vi "AutomaticCalibration.vi"(8 "error in (no error)":errorcluster, 11 "Path":path) -> (0 "error out":errorcluster, 3 "Path Out":path)   [LabVIEW 2013, in "main.lvlib"]
uses:
  main.lvlib
  <vilib>/Analysis/6fits.llb/Curve Fitting Criteria.ctl
  Controls/Enum Save Action Events.ctl
  <vilib>/Analysis/1siggen.llb/Ramp Pattern by Samples.vi
  <userlib>/_OpenG.lib/file/file.llb/File Exists - Scalar__ogtk.vi
  Globals/DataAcqRecordPathGlobal.vi
  <vilib>/Analysis/NI_AAL_SigProc.lvlib
  <vilib>/Analysis/NI_AALBase.lvlib
  <vilib>/Analysis/NI_AALPro.lvlib
panel:
  out "Linear Fit":cluster{dbl[], "Best Linear Fit":dbl[]}[](graph)
  in  "CalibrationCancelBtn":bool
  in  "CalibrationStopBtn":bool
  in  "Slide":dbl(slide) scale=-0.6587369139847334..-0.5375357904577545 scale format="%#_2g"
  out "System XY Graph":cluster{"Ramp Pattern":dbl[], dbl[]}[](graph)
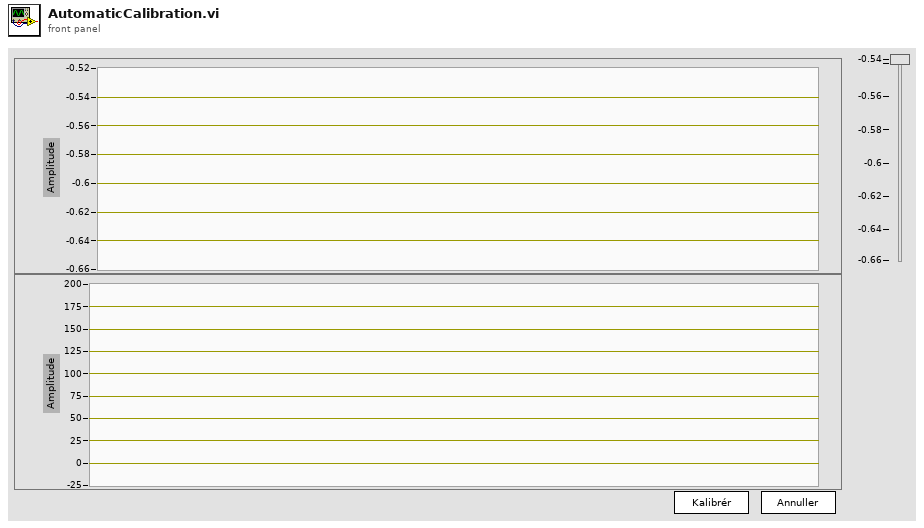
[diagram p1: front panel]
types:
  T1 = typedef "main.lvlib/Enum Save Action Events.ctl" = enum16{"LoadReportPath", "SaveReportPath", "Load Graph Path", "Save Graph Path", "LoadDataPath", "SaveDataPath", "Load Template Path", "Save Template Path", "Load PressureFactor", "Save PressureFactor", "Init", "Load Listbox", "Save Listbox", "LoadHospInfo", "SaveHospInfo", "Load DICOM Activation", "Save DICOM Activation", "LoadDICOMInfoWL", "SaveDICOMInfoWL", "LoadDICOMInfoPACS", "SaveDICOMInfoPACS", "Load ArmCalcMethod", "Save ArmCalcMethod", "LoadItemTags", "SaveItemTags", "LoadDICOMEncoding", "SaveDICOMEncoding", "LoadJournalType", "SaveJournalType", "LoadAcqFilterType", "SaveAcqFilterType", "Load Sequence", "Save Sequence", "Load Acquisition Mode", "Save Acquisition Mode", "Load General Settings", "Save General Settings", "Load Language", "Save Language", "Load Dicom Tags", "Save Dicom Tags", "Load BT Serial", "Save BT Serial", "Load BT License", "Save BT License"}
  T2 = typedef "NI_AALPro.lvlib/Curve Fitting Criteria.ctl" = u16
  T3 = cluster{"Ramp Pattern":dbl[], "Amplitudes":dbl[]}[]
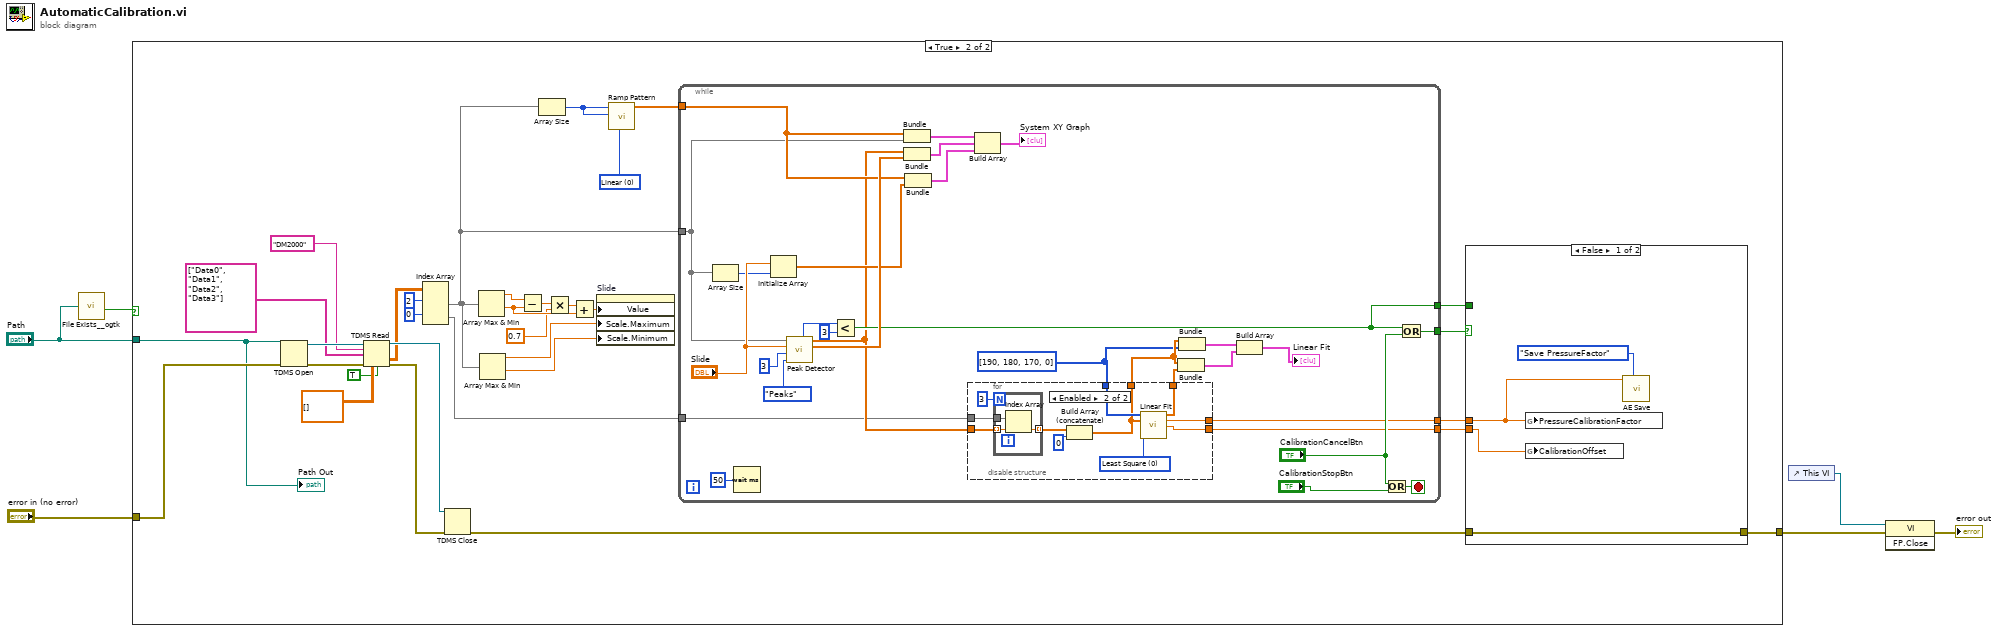
[diagram p0: block diagram]
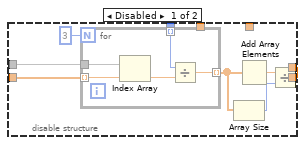
[diagram p3: hidden frame]
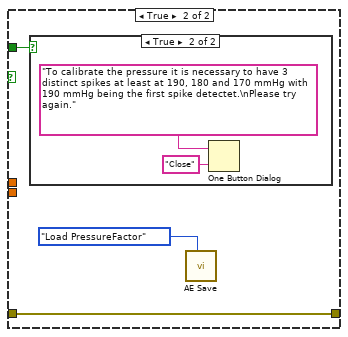
[diagram p4: hidden frame]
diagram:
  n1 = call-poly <userlib>:"File Exists__ogtk.vi"("file path"="Path") -> ("exists"=w4:bool)  [unwired: 6 in, 1 out]
  n2 = case shown="True" w4 {
    tunnel: "error in (no error)" -> [w7 w36]
    tunnel: [w7 w29] -> w2
    tunnel: "Path" -> [_ w28]
    frame False {
    }
    frame True {
      w19 = u16 0 items=["Linear", "Logarithmic"] ("type")
      n3 = TDMS Open(8:w36, 11:w28) -> (0:w38:errorcluster, 3:w39:refnum<k34>)  [unwired: 5 in]
      n4 = TDMS Read(0:w39, 5:"DM2000" ("group name in"), 7:string[] ["Data0", "Data1", "Data2", "Data3"], 11:w38, 12:dbl[][] [], 13:TRUE ("return channels in file order? (F)")) -> (4:w31:refnum<k34>, 10:w18:dbl[][], 15:w32:errorcluster)  [unwired: 2 in, 3 out]
      n5 = Index Array(array=w18, index (row) #1=2 ("index (row)"), index (row) #2=0 ("index (row)")) -> (element #1=w12:dbl[], element #2=w10:dbl[])  [unwired: 2 in]
      n6 = TDMS Close(8:w32, 11:w31) -> (0:w30:errorcluster)  [unwired: 1 out]
      n7 = Array Max & Min(array=w12) -> (max value=w24:dbl, min value=w26:dbl)  [unwired: 2 out]
      n8 = Array Max & Min(array=w12) -> (max value=w15:dbl, min value=w14:dbl)  [unwired: 2 out]
      n9 = Subtract(x=w24, y=w26) -> (x-y=w25:dbl)
      n10 = Array Size(array=w12) -> (size(s)=w20:i32)
      n11 = Multiply(x=w25, y=0.7) -> (x*y=w17:dbl)
      n12 = Add(x=w17, y=w26) -> (x+y=w16:dbl)
      n13 = property on="Slide" class="Slide (strict)"("Value"=w16, "Scale.Maximum"=w15, "Scale.Minimum"=w14) -> ()  [unwired: 2 in, 2 out]
      n14 = call-poly <vilib>:"Ramp Pattern.vi"("type"=w19, "end"=w20, "samples"=w20) -> ("Ramp Pattern"=w13:dbl[])  [unwired: 7 in, 1 out]
      n15 = while {
        tunnel: [w54] -> w33
        tunnel: [w46] -> w27
        tunnel: w13 -> [w59]
        tunnel: w12 -> [w55]
        tunnel: w10 -> [w48]
        tunnel: [w47] -> w11
        tunnel: [w50] -> w8
        stop <- w53 stop-if-true
        w40 = i32[] [190, 180, 170, 0]
        n16 = Array Size(array=w55) -> (size(s)=w56:i32)
        n17 = Wait (ms)(milliseconds to wait=u32 50) -> ()  [unwired: 1 out]
        n18 = Initialize Array("Slide", w56) -> (w62:dbl[])
        n19 = call <vilib>:"Peak Detector.vi"("peaks/valleys"=enum32{"Peaks", "Valleys"}."Peaks", "width"=3, "threshold"="Slide", "X"=w55) -> ("Amplitudes"=w65:dbl[], "Locations"=w49:dbl[], "# found"=w67:i32)  [unwired: 3 in, 2 out]
        n20 = Less?(x=w67, y=3) -> (x < y?=w50:bool)
        n21 = Bundle("Ramp Pattern"=w59, w55) -> (w58:cluster{"Ramp Pattern":dbl[], dbl[]})  [unwired: 1 in]
        n22 = Bundle("Locations"=w49, "Amplitudes"=w65) -> (w63:cluster{"Locations":dbl[], "Amplitudes":dbl[]})  [unwired: 1 in]
        n23 = Bundle("Ramp Pattern"=w59, w62) -> (w57:cluster{"Ramp Pattern":dbl[], dbl[]})  [unwired: 1 in]
        n24 = disable-structure shown="Enabled" {
          disable-tunnel: [w76 w89] -> w47
          disable-tunnel: w48 -> [w75 w93]
          disable-tunnel: w49 -> [w74 w92]
          disable-tunnel: w40 -> [w70 w91]
          disable-tunnel: [_ w87] -> w46
          disable-tunnel: [_ w84] -> w45
          disable-tunnel: [_ w83] -> w41
          frame Disabled {
            n25 = for {
              N: 3 -> [_]
              tunnel: w74 -> [w82] mode=indexing
              tunnel: w75 -> [w81]
              tunnel: [w80] -> w73 mode=indexing
              tunnel: w70 -> [w78] mode=indexing
              n26 = Index Array(array=w81, index=w82) -> (element=w79:dbl)
              n27 = Divide(x=w78, y=w79) -> (x/y=w80:dbl)
            }
            n28 = Array Size(array=w73) -> (size(s)=w72:i32)
            n29 = Add Array Elements(numeric array=w73) -> (sum=w77:dbl)
            n30 = Divide(x=w77, y=w72) -> (x/y=w76:dbl)
          }
          frame Enabled {
            w90 = T2 0 items=["Least Square", "Least Absolute Residual", "Bisquare"] ("method")
            n31 = for {
              N: 3 -> [_]
              tunnel: w92 -> [w96] mode=indexing
              tunnel: w93 -> [w95]
              tunnel: [w94] -> w86 mode=indexing
              n32 = Index Array(array=w95, index=w96) -> (element=w94:dbl)
            }
            n33 = Build Array (concatenate)(w86, 0) -> (w83:dbl[])
            n34 = call <vilib>:"Linear Fit.vi"("Y"=w91, "X"=w83, "method"=w90) -> ("Best Linear Fit"=w84:dbl[], "slope"=w89:dbl, "intercept"=w87:dbl)  [unwired: 8 in, 2 out]
          }
        }
        n35 = Build Array(w58, w63, w57) -> (→"System XY Graph":T3)
        n36 = Bundle(w41, "Best Linear Fit"=w45) -> (w43:cluster{dbl[], "Best Linear Fit":dbl[]})  [unwired: 1 in]
        n37 = Bundle(w41, w40) -> (w44:cluster{dbl[], i32[]})  [unwired: 1 in]
        n38 = Build Array(w44, w43) -> (→"Linear Fit":cluster{dbl[], "Best Linear Fit":dbl[]}[])
        n39 = Or(x="CalibrationCancelBtn", y="CalibrationStopBtn") -> (x .or. y?=w53:bool)
        n40 = Or(x=w50, y="CalibrationCancelBtn") -> (x .or. y?=w54:bool)
      }
      n41 = case shown="False" w33 {
        tunnel: w27 -> [w98 _]
        tunnel: [w99 w103] -> w29
        tunnel: w30 -> [w99 w103]
        tunnel: w11 -> [w97 _]
        tunnel: w8 -> [_ w102]
        frame False {
          n42 = global write "DataAcqRecordPathGlobal.vi" "PressureCalibrationFactor"(w97) -> ()
          n43 = global write "DataAcqRecordPathGlobal.vi" "CalibrationOffset"(w98) -> ()
          n44 = call "AE Save.vi"("Variant In"=w97, "Action"=Enum_Save_Action_Events."Save PressureFactor") -> ()  [unwired: 7 in, 2 out]
        }
        frame True {
          n45 = case shown="True" w102 {
            frame False {
            }
            frame True {
              n46 = One Button Dialog(message="To calibrate the pressure it is necessary to have 3 distinct spikes at least at 190, 180 and 170 mmHg with 190 mmHg being the first spike detectet.\nPlease try again.", button name ("OK")="Close") -> ()  [unwired: 1 out]
            }
          }
          n47 = call "AE Save.vi"("Action"=Enum_Save_Action_Events."Load PressureFactor") -> ()  [unwired: 8 in, 2 out]
        }
      }
      "Path Out" <- w28
    }
  }
  n48 = control-ref of="This VI"() -> (w1:refnum<vi>)
  n49 = invoke class="VI" method="FP.Close"(reference=w1, error in=w2) -> (error out=→"error out":errorcluster)  [unwired: 1 in, 2 out]
